vi "piezoDoubleWriteWrite.vi"(1 "mode":u16(ring) items=["fractional", "position", "voltage"], 2 "piezo2":dbl, 3 "piezo1":dbl) -> ()   [LabVIEW 2017]
uses:
  <vilib>/DAQmx/write.llb/DAQmx Write (Analog 1D DBL NChan 1Samp).vi
  globalDevices.vi
  <vilib>/DAQmx/miscellaneous.llb/DAQmx Fill In Error Info.vi
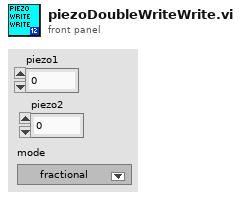
[diagram p1: front panel]
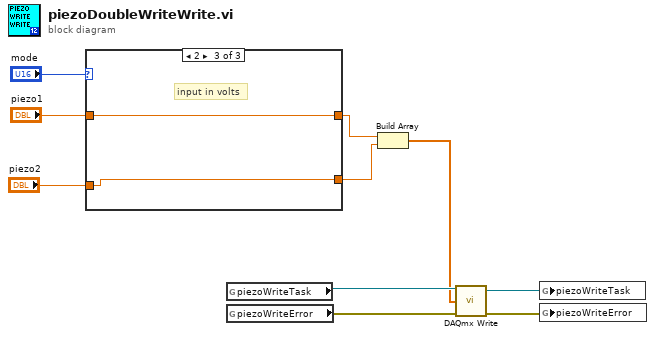
[diagram p0: block diagram]
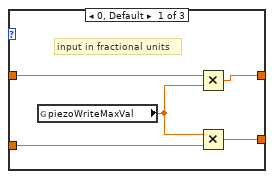
[diagram p2: hidden frame]
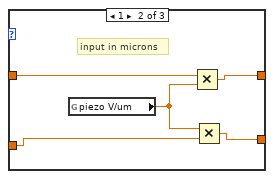
[diagram p3: hidden frame]
diagram:
  n1 = case shown="2" "mode" {
    tunnel: "piezo1" -> [w15 w20 w22]
    tunnel: [w14 w19 w22] -> w3
    tunnel: "piezo2" -> [w13 w18 w21]
    tunnel: [w11 w16 w21] -> w2
    frame 0, Default {
      # "input in fractional units"
      n2 = global read "globalDevices.vi" "piezoWriteMaxVal"() -> (w12:dbl)
      n3 = Multiply(x=w15, y=w12) -> (x*y=w14:dbl)
      n4 = Multiply(x=w12, y=w13) -> (x*y=w11:dbl)
    }
    frame 1 {
      # "input in microns"
      n5 = global read "globalDevices.vi" "piezo V/um"() -> (w17:dbl)
      n6 = Multiply(x=w20, y=w17) -> (x*y=w19:dbl)
      n7 = Multiply(x=w17, y=w18) -> (x*y=w16:dbl)
    }
    frame 2 {
      # "input in volts"
    }
  }
  n8 = global read "globalDevices.vi" "piezoWriteTask"() -> (w10:refnum<k21>)
  n9 = global read "globalDevices.vi" "piezoWriteError"() -> (w9:errorcluster)
  n10 = Build Array(w3, w2) -> (w1:dbl[])
  n11 = call-poly <vilib>:"DAQmx Write.vi"("task/channels in"=w10, "data"=w1, "error in"=w9) -> ("task out"=w6:refnum<k21>, "error out"=w5:errorcluster)  [unwired: 10 in, 1 out]
  n12 = global write "globalDevices.vi" "piezoWriteTask"(w6) -> ()
  n13 = global write "globalDevices.vi" "piezoWriteError"(w5) -> ()
